vi "Execute.vi"(8 "error in (no error)":errorcluster, 10 "UserEvents in":refnum<class "UserEvents.lvclass">, 11 "Controller in":refnum<class "Controller.lvclass">) -> (0 "error out":errorcluster, 3 "Controller out":refnum<class "Controller.lvclass">)   [LabVIEW 2015, in "Controller.lvclass"]
uses:
  Controller.lvclass
  Typedefs/State Types.ctl
  Typedefs/FAMT Typedefs.lvlib
  Commands/Command/Command.lvclass
  Context/Context.lvclass
  Model/Model/Model.lvclass
  UserEvents/UserEvents.lvclass
  Model/Boot Loader/Boot Loader.lvclass
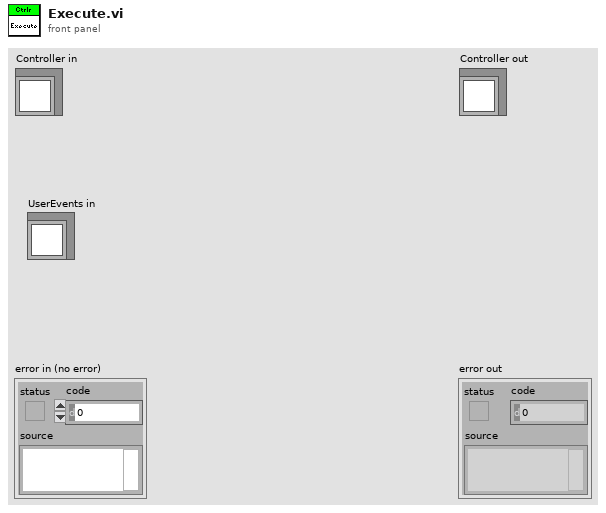
[diagram p1: front panel]
types:
  T1 = typedef "FAMT Typedefs.lvlib/State Types.ctl" = enum16{"Offline State", "Fault State", "Standby State", "Disabled State", "Enabled State", "Wait For User Input State", "Perform Scan State"}
  T2 = typedef "FAMT Typedefs.lvlib/Subscribe Data Events.ctl" = cluster{"Command":refnum<user-event>}
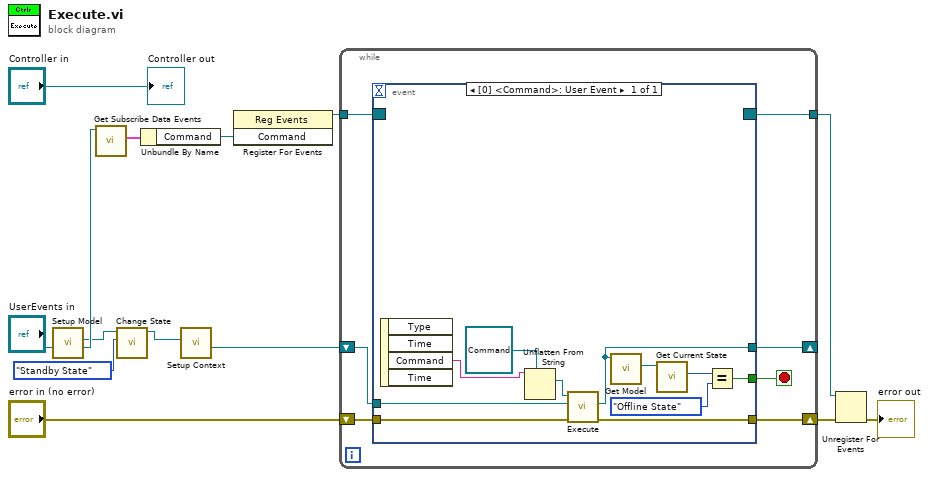
[diagram p0: block diagram]
diagram:
  n1 = call "Setup Model.vi"("User Events in"="UserEvents in") -> ("User Events out"=w6:refnum<class "UserEvents.lvclass">, "Model out"=w5:refnum<class "Model.lvclass">)  [unwired: 7 in, 2 out]
  n2 = call "Get Subscribe Data Events.vi"("UserEvents in"=w6) -> ("Subscribe Data Events"=w13:T2)  [unwired: 9 in, 1 out]
  n3 = call "Change State.vi"("State Types"=State_Types."Standby State" ("State:"), "Model in"=w5) -> ("Model out"=w4:refnum<class "Model.lvclass">)  [unwired: 8 in, 1 out]
  n4 = Unbundle By Name(w13) -> ("Command"=w9:refnum<user-event>)
  n5 = call "Setup Context.vi"("Model in"=w4) -> ("Context out"=w3:refnum<class "Context.lvclass">)  [unwired: 8 in, 2 out]
  n6 = register-events(w9) -> (reference out=w12:refnum<event-registration>)  [unwired: 2 in, 1 out]
  n7 = while {
    shift-right: [w20] -> w10
    shift-left: "error in (no error)" -> [w17]
    shift-right: [w19] -> _
    shift-left: w3 -> [w21]
    tunnel: w12 -> [w16]
    tunnel: [w15] -> w11
    stop <- w18 stop-if-true
    n8 = event shown="[0] <Command>: User Event" {
      selector: w16 -> [_]
      dyn-events: [_] -> w15
      timeout: _ -> [_]
      tunnel: w21 -> [w30]
      tunnel: [w27] -> w20
      tunnel: [w26] -> w19
      tunnel: [w25] -> w18
      tunnel: w17 -> [w23]
      event User Event {
        n9 = event-data() -> ("Command"=w22:string)  [unwired: 1 in, 3 out]
        n10 = Unflatten From String(type=refnum<class "Command.lvclass"> refnum ("Command.lvclass"), binary string=w22) -> (value=w31:refnum<class "Command.lvclass">)  [unwired: 3 in, 2 out]
        n11 = call-dynamic "Execute.vi"("error in (no error)"=w23, "Context in"=w30, "Command in"=w31) -> ("error out"=w27:errorcluster, "Context out"=w26:refnum<class "Context.lvclass">)  [unwired: 6 in, 1 out]
        n12 = call "Get Model.vi"("Context in"=w26) -> ("Model"=w29:refnum<class "Model.lvclass">)  [unwired: 9 in, 1 out]
        n13 = call "Get Current State.vi"("Model in"=w29) -> ("State Types"=w24:T1)  [unwired: 9 in, 1 out]
        n14 = Equal?(x=w24, y=State_Types."Offline State") -> (x = y?=w25:bool)
      }
    }
  }
  n15 = Unregister For Events(event registration refnum=w11, error in=w10) -> (error out=→"error out":errorcluster)
  "Controller out" <- "Controller in"
